vi "Single Channel Search for Property.vi"() -> ()   [LabVIEW 2025]
uses:
  NationalInstruments.VeriStand.SystemDefinitionAPI
  NationalInstruments.VeriStand.SystemStorage
  <vilib>/NI/NI VeriStand Advanced SysDef API/SysDef API/Advanced System Definition.lvlib
panel:
  out "nodePath":string
  out "GetAllPropertiesWithType":string[](array[string])
  out "Array 2":string[](array[string])
  out "Array":string[](array[string])
  in  "System Definition File Path":path=path "C:/Users/Nick/Desktop/VCOM Config System Definition Utility/VeriStand Example Project/Example Project/Example Project.nivssdf"
  out "error out":errorcluster
  in  "error in (no error)":errorcluster
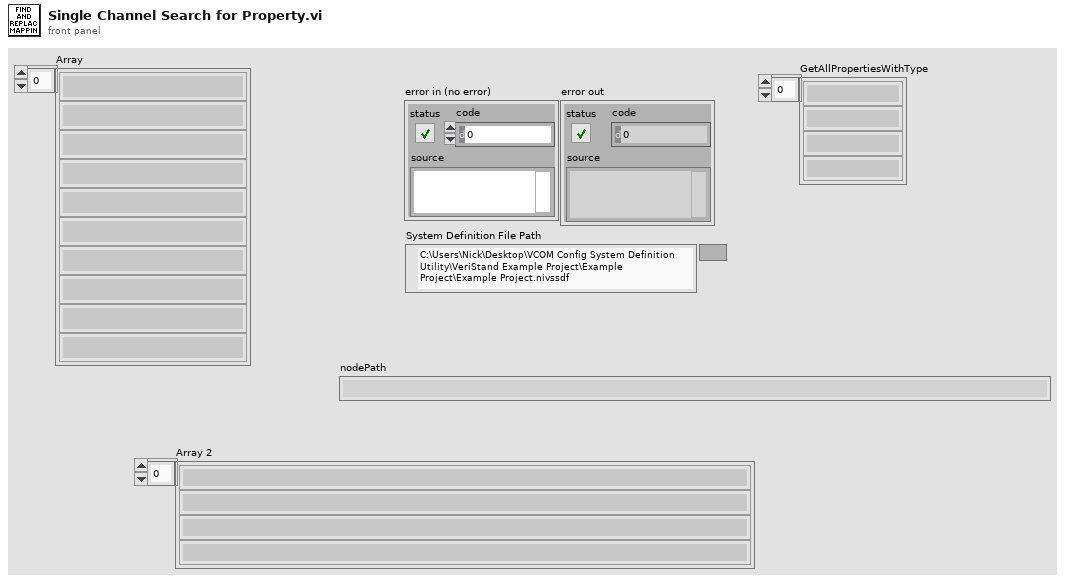
[diagram p1: front panel]
types:
  T1 = typedef "Custom Device API.lvlib/Custom Device Pointer.ctl" = refnum<k24>
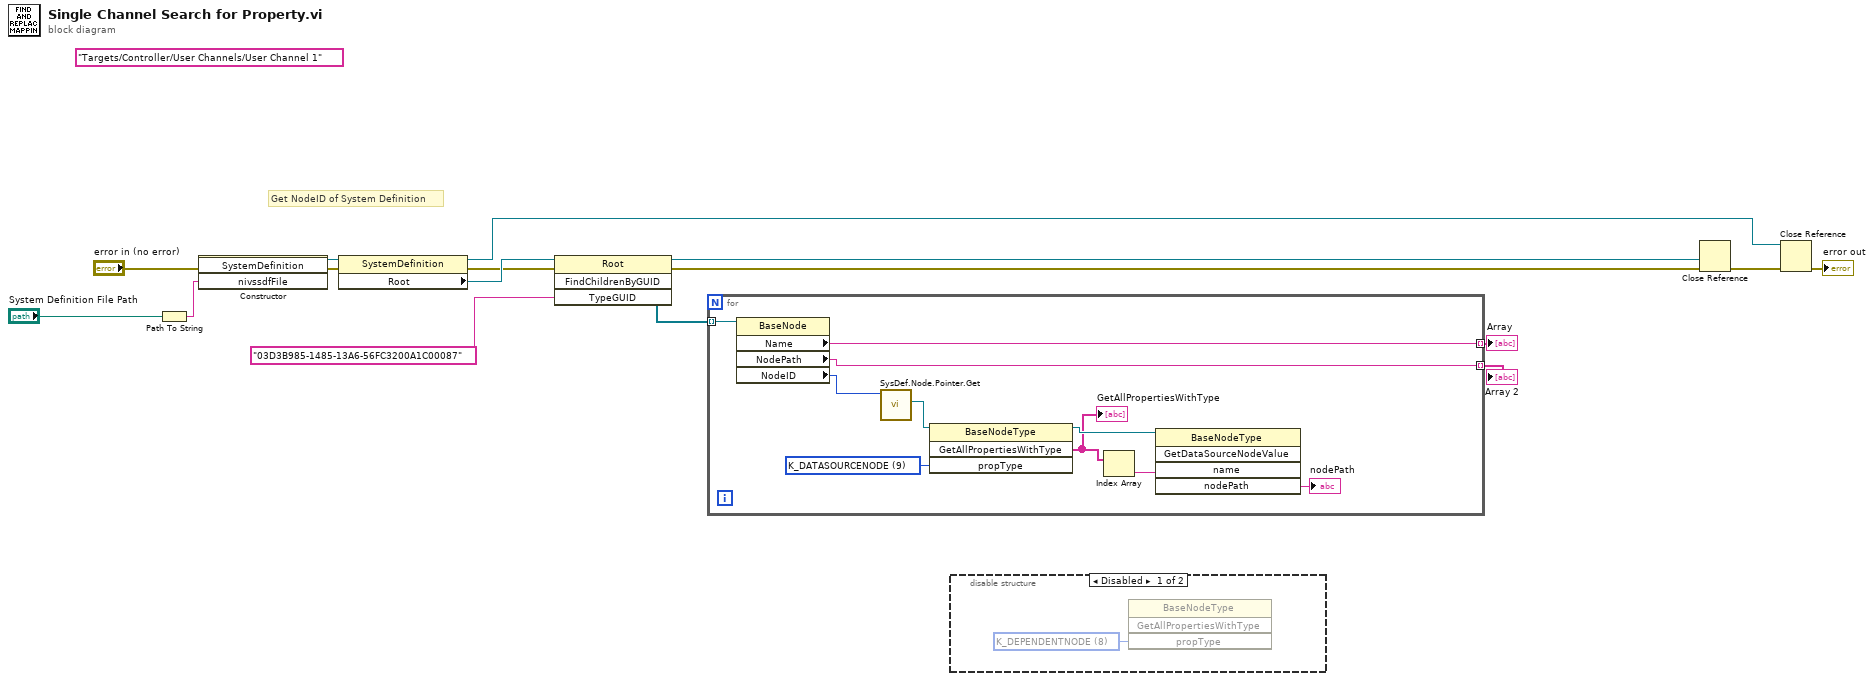
[diagram p0: block diagram]
diagram:
  (unwired) "Targets/Controller/User Channels/User Channel 1" ("TypeGUID")
  # "Get NodeID of System Definition"
  n1 = Path To String(path="System Definition File Path") -> (string=w16:string)
  n2 = constructor class="SystemDefinition"(error in="error in (no error)", "nivssdfFile"=w16) -> (reference out=w14:refnum<k24>, error out=w15:errorcluster)  [unwired: 2 in, 2 out]
  n3 = property class="SystemDefinition"(reference=w14, error in=w15) -> (reference out=w11:refnum<k24>, error out=w7:errorcluster, "Root"=w9:refnum<k24>)
  n4 = invoke class="Root" method="FindChildrenByGUID"(reference=w9, error in=w7, "TypeGUID"="03D3B985-1485-13A6-56FC3200A1C00087") -> (reference out=w6:refnum<k24>, error out=w5:errorcluster, "FindChildrenByGUID"=w4:refnum<k24>[])  [unwired: 1 in, 1 out]
  n5 = for {
    tunnel: w4 -> [w26] mode=indexing
    tunnel: [w25] -> w3 mode=indexing
    tunnel: [w24] -> w1 mode=indexing
    w22 = 9 items=["K_STRING", "K_BOOL", "K_I32", "K_U32", "K_DOUBLE", "K_U64", "K_VARIANT", "K_DEPENDENTFILE", "K_DEPENDENTNODE", "K_DATASOURCENODE", "K_U16", "K_DBLARR", "K_U32ARR", "K_I32ARR", "K_STRINGARR", "K_DICTIONARY", "K_DICTIONARYARR", "K_BINARYSTRING", "K_I16", "K_I64", "K_BOOLARR", "K_U64ARR", "K_U16ARR", "K_I64ARR", "K_I16ARR"] ("propType")
    n6 = property class="BaseNode"(reference=w26) -> ("Name"=w25:string, "NodePath"=w24:string, "NodeID"=w23:u64)  [unwired: 1 in, 2 out]
    n7 = call <vilib>:"SysDef.Node.Pointer.Get.vi"("nodeID"=w23) -> ("Node Pointer"=w21:T1)  [unwired: 7 in, 3 out]
    n8 = invoke class="BaseNodeType" method="GetAllPropertiesWithType"(reference=w21, "propType"=w22) -> (reference out=w20:T1, "GetAllPropertiesWithType"=w19:string[])  [unwired: 2 in, 2 out]
    "GetAllPropertiesWithType" <- w19
    n9 = Index Array(array=w19) -> (element=w18:string)  [unwired: 1 in]
    n10 = invoke class="BaseNodeType" method="GetDataSourceNodeValue"(reference=w20, "name"=w18) -> ("nodePath"=→"nodePath":string)  [unwired: 3 in, 4 out]
  }
  "Array" <- w3
  "Array 2" <- w1
  n11 = disable-structure shown="Disabled" {
    frame Disabled {
      w27 = 8 items=["K_STRING", "K_BOOL", "K_I32", "K_U32", "K_DOUBLE", "K_U64", "K_VARIANT", "K_DEPENDENTFILE", "K_DEPENDENTNODE", "K_DATASOURCENODE", "K_U16", "K_DBLARR", "K_U32ARR", "K_I32ARR", "K_STRINGARR", "K_DICTIONARY", "K_DICTIONARYARR", "K_BINARYSTRING", "K_I16", "K_I64", "K_BOOLARR", "K_U64ARR", "K_U16ARR", "K_I64ARR", "K_I16ARR"] ("propType")
      n12 = invoke class="BaseNodeType" method="GetAllPropertiesWithType"("propType"=w27) -> ()  [unwired: 3 in, 4 out]
    }
    frame Enabled {
    }
  }
  n13 = Close Reference(reference=w6, error in (no error)=w5) -> (error out=w8:errorcluster)
  n14 = Close Reference(reference=w11, error in (no error)=w8) -> (error out=→"error out":errorcluster)
